vi "15_HighRes.vi"(8 "error in\n(no error)":errorcluster) -> (0 "error out":errorcluster)   [LabVIEW 2014]
uses:
  SwabianInstruments.TimeTagger
panel:
  out "error message":string
  out "Mean value and RMS":dbl[][](graph)
  in  "Start TimeDifferences\nmeasurement":bool
  out "TimeDifferences data (only 40 out of 5000 bins)":i32[][](graph)
  in  "stop":bool
  in  "click_channel":i32(ring) items=["1 (Standard)"=1, "2 (Standard)"=2, "3 (Standard)"=3, "4 (Standard)"=4, "5 (Standard)"=5, "6 (Standard)"=6, "7 (Standard)"=7, "8 (Standard)"=8, "9 (Standard)"=9, "10 (Standard)"=10, "11 (Standard)"=11, "12 (Standard)"=12, "13 (Standard)"=13, "14 (Standard)"=14, "15 (Standard)"=15, "16 (Standard)"=16, "17 (Standard)"=17, "18 (Standard)"=18]
  in  "start_channel":i32(ring) items=["1 (Standard)"=1, "2 (Standard)"=2, "3 (Standard)"=3, "4 (Standard)"=4, "5 (Standard)"=5, "6 (Standard)"=6, "7 (Standard)"=7, "8 (Standard)"=8, "9 (Standard)"=9, "10 (Standard)"=10, "11 (Standard)"=11, "12 (Standard)"=12, "13 (Standard)"=13, "14 (Standard)"=14, "15 (Standard)"=15, "16 (Standard)"=16, "17 (Standard)"=17, "18 (Standard)"=18]
  in  "resolution":i32(ring) items=["Standard", "HighResA", "HighResB", "HighResC"]
  # "This example works only with a Time Tagger Ultra\nand a HighRes license.\n\n- Select a resolution -> the Time Tagger re-connects\n- Select channels to compare and start measurement\n- The Time Differences measurement will acquire 500\n   histograms, each containing 40,000 events generated\n   by the internal test signal (~50 ms per histogram)"
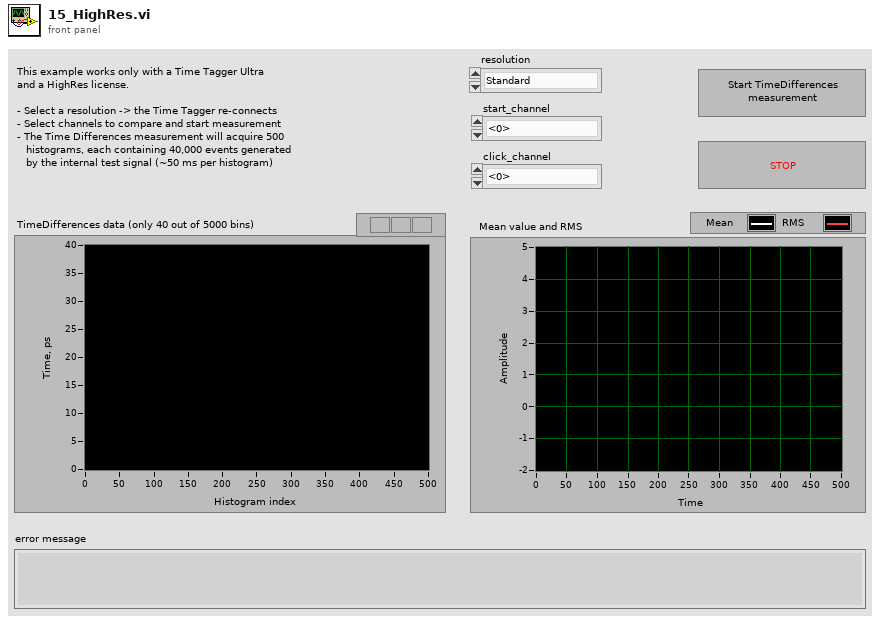
[diagram p1: front panel]
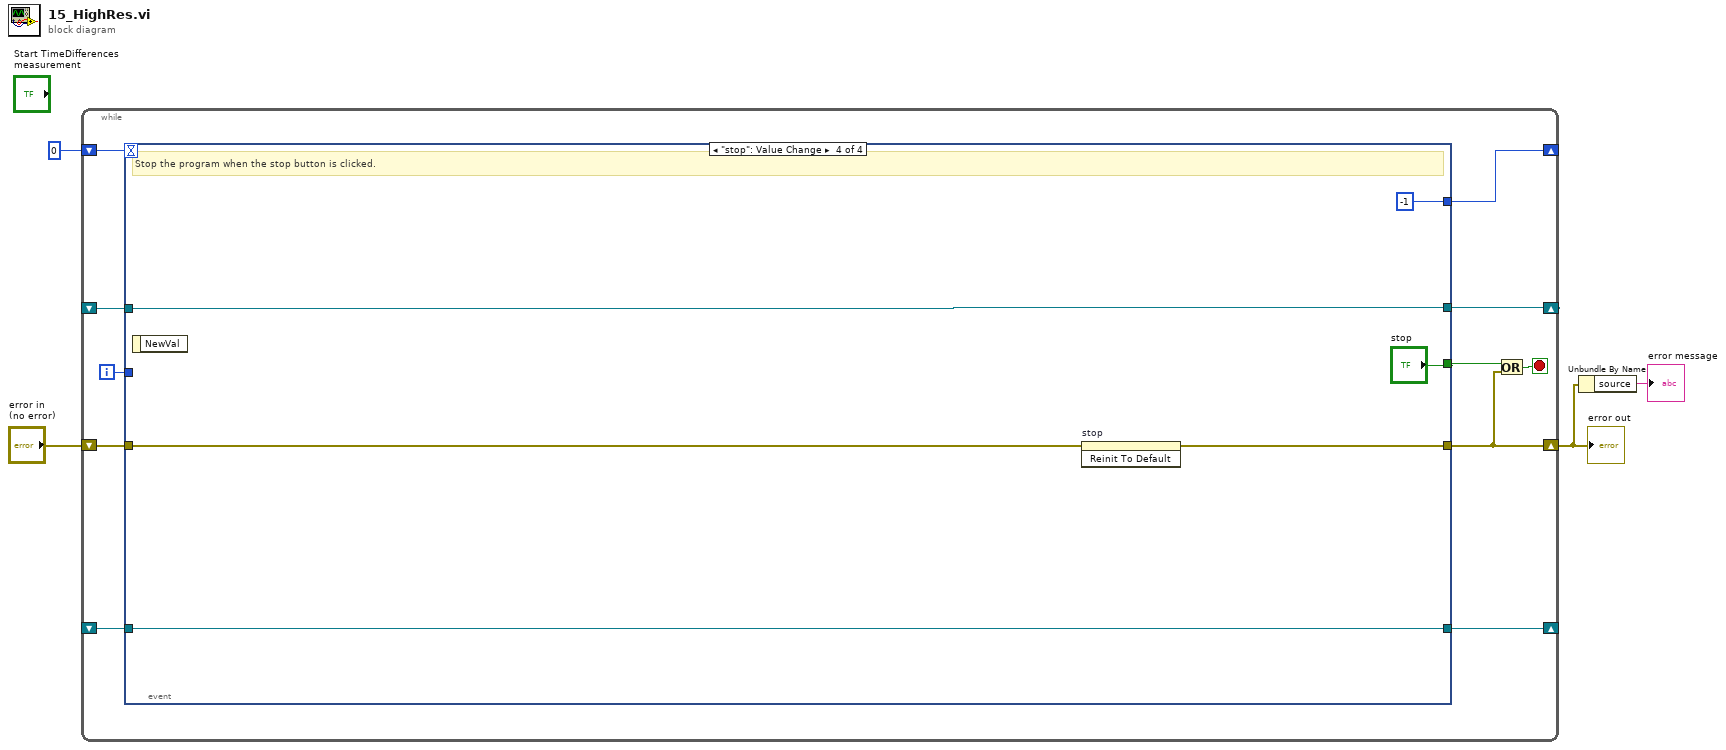
[diagram p0: block diagram]
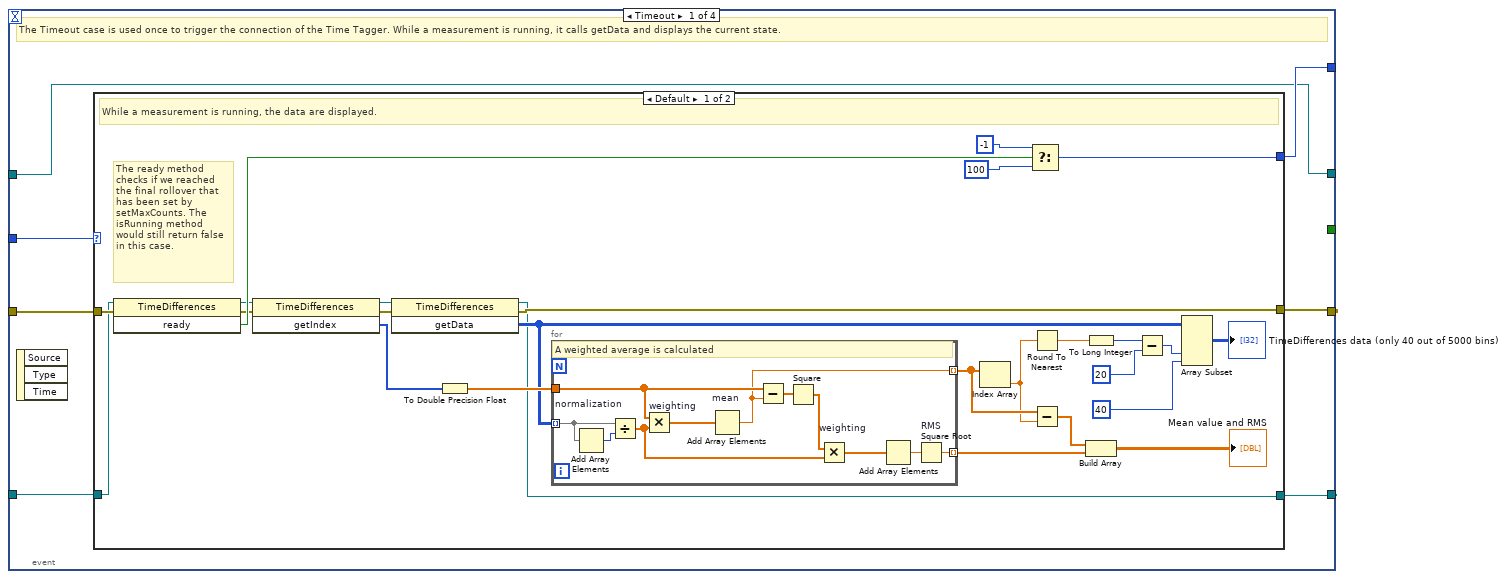
[diagram p2: hidden frame]
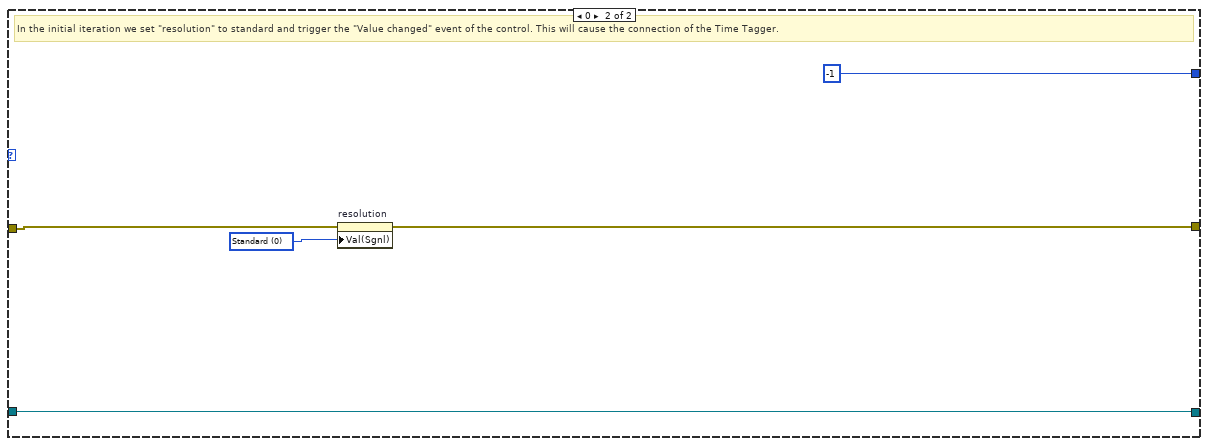
[diagram p3: hidden frame]
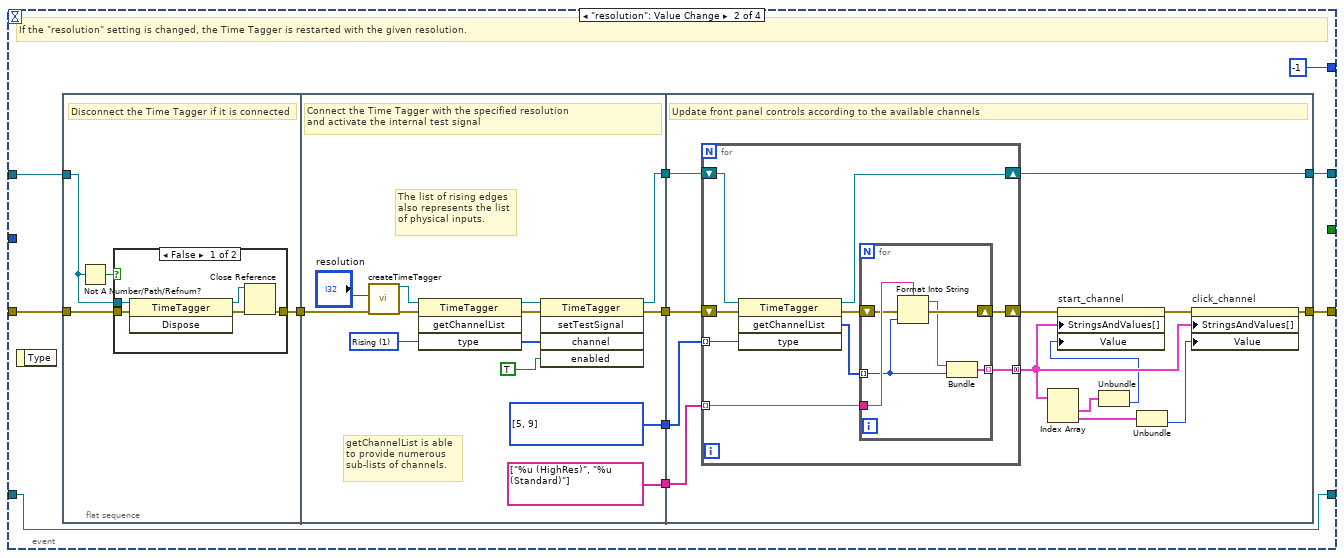
[diagram p4: hidden frame]
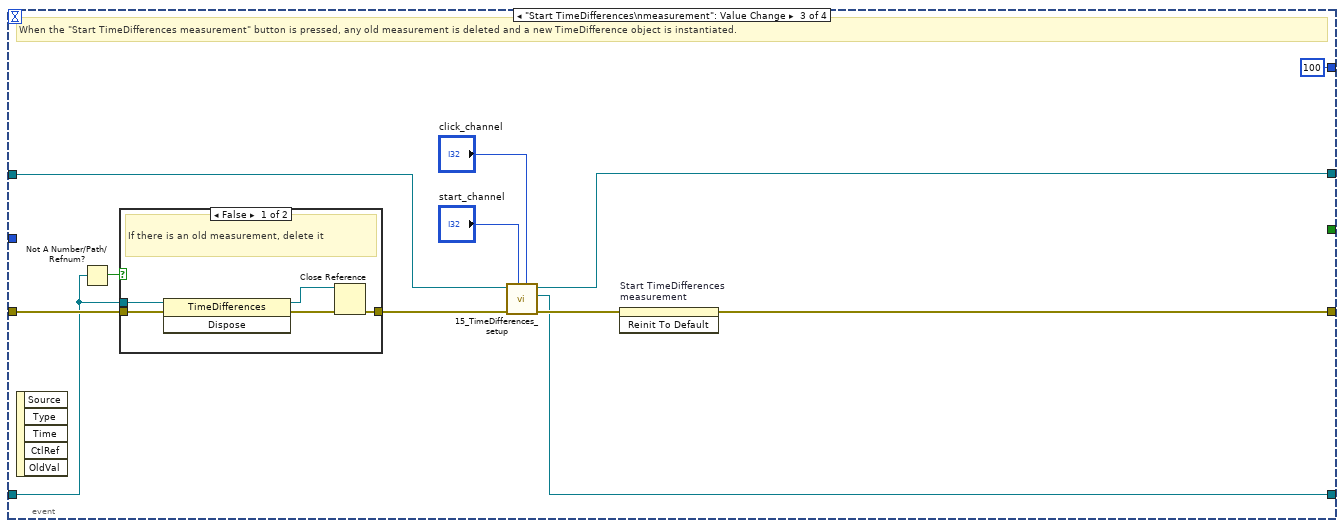
[diagram p6: hidden frame]
diagram:
  n1 = while {
    shift-right: [w15] -> _
    shift-left: _ -> [w14]
    shift-right: [w6] -> w2
    shift-left: "error in\n(no error)" -> [w13]
    shift-right: [w7] -> _
    shift-left: 0 -> [w12]
    shift-right: [w10] -> _
    shift-left: _ -> [w9]
    i -> [w11]
    stop <- w8 stop-if-true
    n2 = event shown="[3] \"stop\": Value Change" {
      selector: _ -> [_ _ _ _]
      dyn-events: _ -> [_ _ _ _]
      timeout: w12 -> [_ _ _ _]
      tunnel: [w16 w68 w127 w149] -> w15
      tunnel: w14 -> [w16 w69 w131 w149]
      tunnel: [_ _ _ "stop"] -> w5
      tunnel: [w20 w74 w137 w145] -> w6
      tunnel: w13 -> [w21 w71 w133 w146]
      tunnel: w11 -> [w22 _ _ _]
      tunnel: [w17 -1 100 -1 ("f")] -> w7
      tunnel: [w18 w65 w130 w150] -> w10
      tunnel: w9 -> [w19 w65 w129 w150]
      event Timeout {
        # "The Timeout case is used once to trigger the connection of the Time Tagger. While a measurement is running, it calls getData and displays the current state."
        n3 = event-data() -> ()  [unwired: 1 in, 3 out]
        n4 = case shown="Default" w22 {
          tunnel: w21 -> [w48 w63]
          tunnel: [w46 w60] -> w20
          tunnel: w19 -> [w23 w61]
          tunnel: [w43 -1] -> w17
          tunnel: [w24 w61] -> w18
          frame Default {
            # "The ready method\nchecks if we reached\nthe final rollover that\nhas been set by\nsetMaxCounts. The\nisRunning method\nwould still return false\nin this case."
            # "While a measurement is running, the data are displayed."
            n5 = invoke class="TimeDifferences" method="ready"(reference=w23, error in=w48) -> (reference out=w42:refnum<k24>, error out=w40:errorcluster, "ready"=w47:bool)  [unwired: 1 in]
            n6 = invoke class="TimeDifferences" method="getIndex"(reference=w42, error in=w40) -> (reference out=w41:refnum<k24>, error out=w39:errorcluster, "getIndex"=w38:i64[])  [unwired: 1 in]
            n7 = invoke class="TimeDifferences" method="getData"(reference=w41, error in=w39) -> (reference out=w24:refnum<k24>, error out=w46:errorcluster, "getData"=w30:i32[][])  [unwired: 1 in]
            n8 = To Double Precision Float(number=w38) -> (double precision float=w31:dbl[])
            n9 = for {
              tunnel: w31 -> [w56]
              tunnel: w30 -> [w57] mode=indexing
              tunnel: [w55] -> w29 mode=indexing
              tunnel: [w52] -> w26 mode=indexing
              # "A weighted average is calculated"
              n10 = Add Array Elements(numeric array=w57) -> (sum=w58:i32)
              n11 = Divide "normalization"(x=w57, y=w58) -> (x/y=w54:dbl[])
              n12 = Multiply "weighting"(x=w56, y=w54) -> (x*y=w59:dbl[])
              n13 = Add Array Elements "mean"(numeric array=w59) -> (sum=w55:dbl)
              n14 = Subtract(x=w56, y=w55) -> (x-y=w51:dbl[])
              n15 = Square(x=w51) -> (x^2=w50:dbl[])
              n16 = Multiply "weighting"(x=w50, y=w54) -> (x*y=w49:dbl[])
              n17 = Add Array Elements(numeric array=w49) -> (sum=w53:dbl)
              n18 = Square Root "RMS"(x=w53) -> (sqrt(x)=w52:dbl)
            }
            n19 = Index Array(array=w29) -> (element=w28:dbl)  [unwired: 1 in]
            n20 = Select(t=-1, s=w47, f=100) -> (s? t:f=w43:i32)
            n21 = Round To Nearest(number=w28) -> (nearest integer value=w37:dbl)
            n22 = Subtract(x=w29, y=w28) -> (x-y=w27:dbl[])
            n23 = To Long Integer(number=w37) -> (32bit integer=w35:i32)
            n24 = Build Array(w27, w26) -> (→"Mean value and RMS":dbl[][])
            n25 = Subtract(x=w35, y=20) -> (x-y=w33:i32)
            n26 = Array Subset(array=w30, index (col)=w33, length (col)=40 ("length")) -> (→"TimeDifferences data (only 40 out of 5000 bins)":i32[][])  [unwired: 2 in]
          }
          frame 0 {
            w64 = 0 items=["Standard", "HighResA", "HighResB", "HighResC"] ("resolution")
            # "In the initial iteration we set \"resolution\" to standard and trigger the \"Value changed\" event of the control. This will cause the connection of the Time Tagger."
            n27 = property on="resolution" class="Ring (strict)"(error in=w63, "Val(Sgnl)"=w64) -> (error out=w60:errorcluster)  [unwired: 1 in, 1 out]
          }
        }
      }
      event "resolution": Value Change {
        # "If the \"resolution\" setting is changed, the Time Tagger is restarted with the given resolution."
        n28 = event-data() -> ()  [unwired: 1 in, 1 out]
        n29 = flat-sequence {
          tunnel: w71 -> [w79]
          tunnel: [w78] -> w70
          tunnel: w69 -> [w77]
          tunnel: [w92] -> w73
          tunnel: [w93] -> w72
          tunnel: w70 -> [w91]
          tunnel: [string[] ["%u (HighRes)", "%u (Standard)"]] -> w67
          tunnel: [w86] -> w66
          tunnel: [w106] -> w74
          tunnel: [w103] -> w68
          tunnel: w73 -> [w105]
          tunnel: w72 -> [w104]
          tunnel: w67 -> [w101]
          tunnel: w66 -> [w99]
          frame #0 {
            # "Disconnect the Time Tagger if it is connected"
            n30 = Not A Number/Path/Refnum?(number/path/refnum=w77) -> (NaN/Path/Refnum?=w76:bool)
            n31 = case shown="False" w76 {
              tunnel: [w84 w85] -> w78
              tunnel: w77 -> [w82 _]
              tunnel: w79 -> [w80 w85]
              frame False {
                n32 = invoke class="TimeTagger" method="Dispose"(reference=w82, error in=w80) -> (reference out=w83:refnum<k24>, error out=w81:errorcluster)  [unwired: 1 in, 1 out]
                n33 = Close Reference(reference=w83, error in (no error)=w81) -> (error out=w84:errorcluster)
              }
              frame True {
              }
            }
          }
          frame #1 {
            w86 = i32[] [5, 9] items=["All"=0, "Rising"=1, "Falling"=2, "HighResAll"=4, "HighResRising"=5, "HighResFalling"=6, "StandardAll"=8, "StandardRising"=9, "StandardFalling"=10]
            w95 = 1 items=["All"=0, "Rising"=1, "Falling"=2, "HighResAll"=4, "HighResRising"=5, "HighResFalling"=6, "StandardAll"=8, "StandardRising"=9, "StandardFalling"=10] ("type")
            # "getChannelList is able\nto provide numerous\nsub-lists of channels."
            # "The list of rising edges\nalso represents the list\nof physical inputs."
            # "Connect the Time Tagger with the specified resolution\nand activate the internal test signal"
            n34 = call "createTimeTagger.vi"("error in (no error)"=w91, "resolution"="resolution") -> ("error out"=w90:errorcluster, "TimeTagger ref out"=w88:refnum<k24>)  [unwired: 8 in]
            n35 = invoke class="TimeTagger" method="getChannelList"(reference=w88, error in=w90, "type"=w95) -> (reference out=w96:refnum<k24>, error out=w97:errorcluster, "getChannelList"=w98:i32[])  [unwired: 1 in, 1 out]
            n36 = invoke class="TimeTagger" method="setTestSignal"(reference=w96, error in=w97, "channel"=w98, "enabled"=TRUE) -> (reference out=w93:refnum<k24>, error out=w92:errorcluster)  [unwired: 1 in, 3 out]
          }
          frame #2 {
            # "Update front panel controls according to the available channels"
            n37 = for {
              tunnel: w99 -> [w120] mode=indexing
              tunnel: w101 -> [w117] mode=indexing
              tunnel: [w114] -> w102 mode=concatenating
              shift-right: [w113] -> w111
              shift-left: w105 -> [w119]
              shift-right: [w112] -> w103
              shift-left: w104 -> [w118]
              n38 = invoke class="TimeTagger" method="getChannelList"(reference=w118, error in=w119, "type"=w120) -> (reference out=w112:refnum<k24>, error out=w116:errorcluster, "getChannelList"=w115:i32[])  [unwired: 1 in, 1 out]
              n39 = for {
                tunnel: w117 -> [w126]
                tunnel: w115 -> [w124] mode=indexing
                tunnel: [w123] -> w114 mode=indexing
                shift-right: [w122] -> w113
                shift-left: w116 -> [w125]
                n40 = Format Into String(format string=w126, error in=w125, w124) -> (resulting string=w121:string, error out=w122:errorcluster)  [unwired: 1 in]
                n41 = Bundle(w121, w124) -> (w123:cluster{string, i32})  [unwired: 1 in]
              }
            }
            n42 = Index Array(array=w102) -> (element #1=w109:cluster{string, i32}, element #2=w108:cluster{string, i32})  [unwired: 2 in]
            n43 = Unbundle(w109) -> (w100:i32)  [unwired: 1 out]
            n44 = property on="start_channel" class="Ring (strict)"(error in=w111, "StringsAndValues[]"=w102, "Value"=w100) -> (error out=w110:errorcluster)  [unwired: 1 in, 1 out]
            n45 = Unbundle(w108) -> (w107:i32)  [unwired: 1 out]
            n46 = property on="click_channel" class="Ring (strict)"(error in=w110, "StringsAndValues[]"=w102, "Value"=w107) -> (error out=w106:errorcluster)  [unwired: 1 in, 1 out]
          }
        }
      }
      event "Start TimeDifferences\nmeasurement": Value Change {
        # "When the \"Start TimeDifferences measurement\" button is pressed, any old measurement is deleted and a new TimeDifference object is instantiated."
        n47 = event-data() -> ()  [unwired: 1 in, 5 out]
        n48 = Not A Number/Path/Refnum?(number/path/refnum=w129) -> (NaN/Path/Refnum?=w134:bool)
        n49 = case shown="False" w134 {
          tunnel: [w143 w144] -> w132
          tunnel: w129 -> [w141 _]
          tunnel: w133 -> [w139 w144]
          frame False {
            # "If there is an old measurement, delete it"
            n50 = invoke class="TimeDifferences" method="Dispose"(reference=w141, error in=w139) -> (reference out=w142:refnum<k24>, error out=w140:errorcluster)  [unwired: 1 in, 1 out]
            n51 = Close Reference(reference=w142, error in (no error)=w140) -> (error out=w143:errorcluster)
          }
          frame True {
          }
        }
        n52 = call "15_TimeDifferences_setup.vi"("click_channel"="click_channel", "start_channel"="start_channel", "error in (no error)"=w132, "TimeTagger ref in"=w131) -> ("error out"=w138:errorcluster, "TimeDifferences ref out"=w130:refnum<k24>, "TimeTagger ref out"=w127:refnum<k24>)  [unwired: 5 in]
        n53 = invoke on="Start TimeDifferences\nmeasurement" class="Bool" method="Reinit To Default"(error in=w138) -> (error out=w137:errorcluster)  [unwired: 2 in, 2 out]
      }
      event "stop": Value Change {
        # "Stop the program when the stop button is clicked."
        n54 = event-data() -> ()  [unwired: 1 in, 1 out]
        n55 = invoke on="stop" class="Bool (strict)" method="Reinit To Default"(error in=w146) -> (error out=w145:errorcluster)  [unwired: 2 in, 2 out]
      }
    }
    n56 = Or(x=w5, y=w6) -> (x .or. y?=w8:bool)
  }
  "error out" <- w2
  n57 = Unbundle By Name(w2) -> ("source"=→"error message":string)
